vi "Configure Hold.vi"(0 "VISA resource name":refnum<visa-resource-name>, 1 "Enable Hold? (T: Enabled)":bool=TRUE, 2 "Window (1.00000 %)":dbl=1.0 format="%_6g", 3 "Count (5)":i32=5, 5 "error in (no error)":errorcluster) -> (14 "VISA resource name out":refnum<visa-resource-name>, 19 "error out":errorcluster)   [LabVIEW 2009, in "Keithley 2000.lvlib"]
doc: "This VI configures the hold function of the instrument. The hold function causes the instrument to wait for a stable reading before returning a reading."
uses:
  <instrlib>/Keithley 2000/Keithley 2000.lvlib
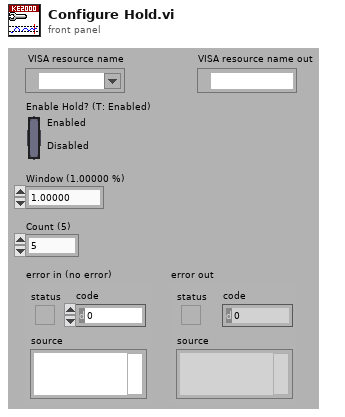
[diagram p1: front panel]
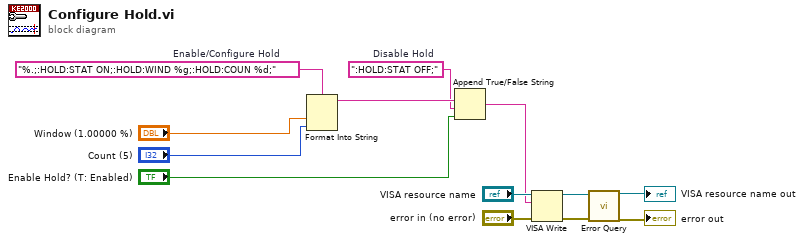
[diagram p0: block diagram]
diagram:
  w6 = ":HOLD:STAT OFF;"  # Disable Hold
  w11 = "%.;:HOLD:STAT ON;:HOLD:WIND %g;:HOLD:COUN %d;"  # Enable/Configure Hold
  n1 = Format Into String(format string=w11, "Window (1.00000 %)", "Count (5)") -> (resulting string=w7:string)  [unwired: 2 in, 1 out]
  n2 = Append True/False String(1:"Enable Hold? (T: Enabled)", 2:w6, 3:w7) -> (0:w5:string)  [unwired: 1 in]
  n3 = VISA Write(VISA resource name="VISA resource name", write buffer=w5, error in (no error)="error in (no error)") -> (VISA resource name out=w4:refnum<visa-resource-name>, error out=w3:errorcluster)  [unwired: 1 out]
  n4 = call <instrlib>:"Error Query.vi"("VISA resource name"=w4, "error in (no error)"=w3) -> ("VISA resource name out"=→"VISA resource name out":refnum<visa-resource-name>, "error out"=→"error out":errorcluster)  [unwired: 14 in, 2 out]
